vi "UpdateDeviceTemperature.vi"(8 "error in (no error)":errorcluster, 11 "fpga reference":refnum<k20>) -> (0 "error out":errorcluster, 1 "valid":bool, 2 "temperature":dbl)   [LabVIEW 2017, in "DeviceHealth.lvlib"]
uses:
  <vilib>/addons/InsightCM/Devices/Shared/Common/DeviceHealth/DeviceHealth.lvlib
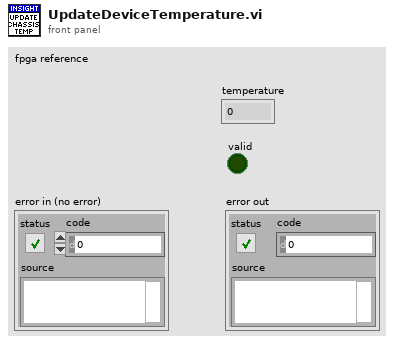
[diagram p1: front panel]
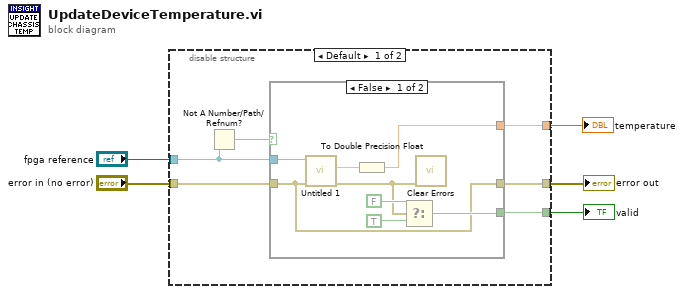
[diagram p0: block diagram]
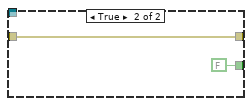
[diagram p2: hidden frame]
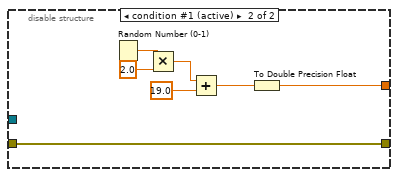
[diagram p3: hidden frame]
diagram:
  n1 = disable-structure shown="Default" {
    disable-tunnel: "error in (no error)" -> [w11 w22]
    disable-tunnel: "fpga reference" -> [w9 _]
    disable-tunnel: [w10 w22] -> w3
    disable-tunnel: [w7 w23] -> w2
    disable-tunnel: [w6 _] -> w1
    frame condition #0 {
      n2 = Not A Number/Path/Refnum?(number/path/refnum=w9) -> (NaN/Path/Refnum?=w8:bool)
      n3 = case shown="False" w8 {
        tunnel: w11 -> [w13 w21]
        tunnel: w9 -> [w15 _]
        tunnel: [w13 w21] -> w10
        tunnel: [w19 _] -> w7
        tunnel: [w16 FALSE] -> w6
        frame False {
          n4 = call <vilib>:"Untitled 1.vi"("error in"=w13, "fpga reference"=w15) -> ("error out"=w14:errorcluster, "Chassis Temperature"=w12:sgl)  [unwired: 8 in]
          n5 = To Double Precision Float(number=w12) -> (double precision float=w19:dbl)
          n6 = Select(t=FALSE, s=w14, f=TRUE) -> (s? t:f=w16:bool)
          n7 = call <vilib>:"Clear Errors.vi"("error in (no error)"=w14) -> ()  [unwired: 5 in, 2 out]
        }
        frame True {
        }
      }
    }
    frame condition #1 (active) {
      n8 = Random Number (0-1)() -> (number: 0 to 1=w27:dbl)
      n9 = Multiply(x=w27, y=2.0) -> (x*y=w25:dbl)
      n10 = Add(x=w25, y=19.0) -> (x+y=w28:dbl)
      n11 = To Double Precision Float(number=w28) -> (double precision float=w23:dbl)
    }
  }
  "error out" <- w3
  "temperature" <- w2
  "valid" <- w1
